vi "ButtonAutoRampStack.vi"(11 "Buttons":bool[](array[boolean])) -> ()   [LabVIEW 2014]
uses:
  LowerLiftAndOpenArms.ctl
  AutomationGlobals.vi
  ToteCount.vi
  Gantry/GantryGlobals.vi
panel:
  in  "Buttons 4":bool[](array[boolean])
  in  "Buttons 3":bool[](array[boolean])
  in  "Buttons 2":bool[](array[boolean])
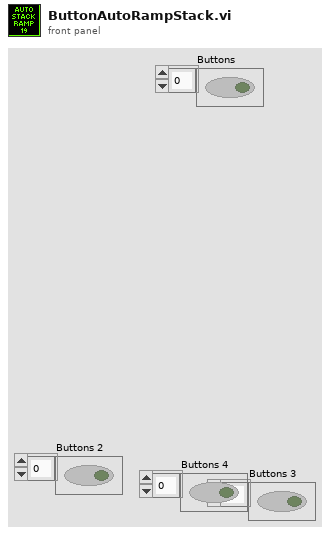
[diagram p1: front panel]
types:
  T1 = typedef "LowerLiftAndOpenArms.ctl" = enum16{"WaitingForInput", "LowerLift", "OpenArms", "LowerLiftMore", "CloseArms", "RaiseLift", "StopArms"}
  T2 = typedef "WPI_SwitchDevRef.ctl" = cluster{"DevStatus":errorcluster, "DIO Channel":T3, "Controller":T4, "CntIndex":T5, "Normally Closed":bool}
  T3 = typedef "FPGA_DIOChannel.ctl" = enum8{"DIO 0", "DIO 1", "DIO 2", "DIO 3", "DIO 4", "DIO 5", "DIO 6", "DIO 7", "DIO 8", "DIO 9", "DIO MXP 0", "DIO MXP 1", "DIO MXP 2", "DIO MXP 3", "DIO MXP 4", "DIO MXP 5", "DIO MXP 6", "DIO MXP 7", "DIO MXP 8", "DIO MXP 9", "DIO MXP 10", "DIO MXP 11", "DIO MXP 12", "DIO MXP 13", "DIO MXP 14", "DIO MXP 15", "Invalid"}
  T4 = typedef "FPGA_TypedefDigitalModule.ctl" = enum16{"Controller 1"}
  T5 = typedef "FPGA_CounterCtrSystemIndex.ctl" = enum8{"Ctr 0", "Ctr 1", "Ctr 2", "Ctr 3", "Ctr 4", "Ctr 5", "Ctr 6", "Ctr 7", "Invalid"}
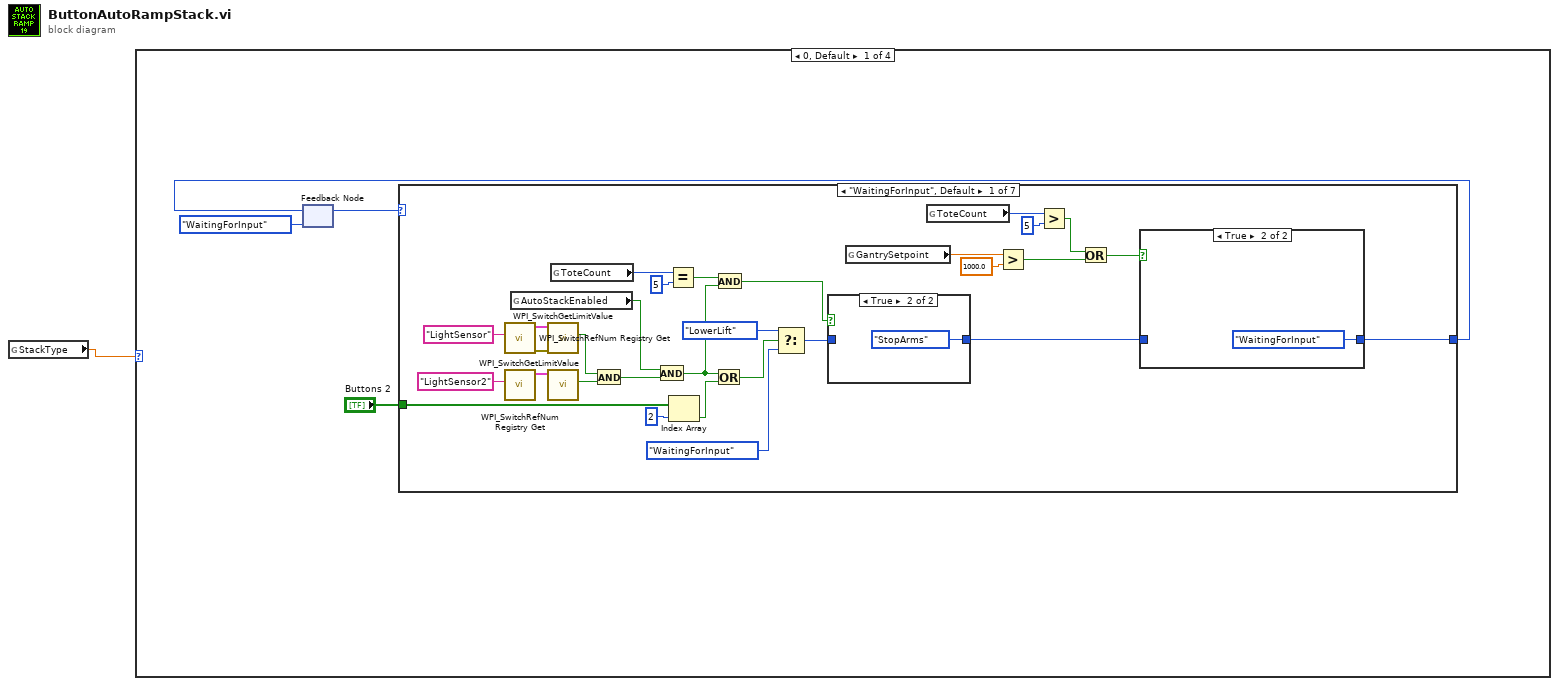
[diagram p0: block diagram]
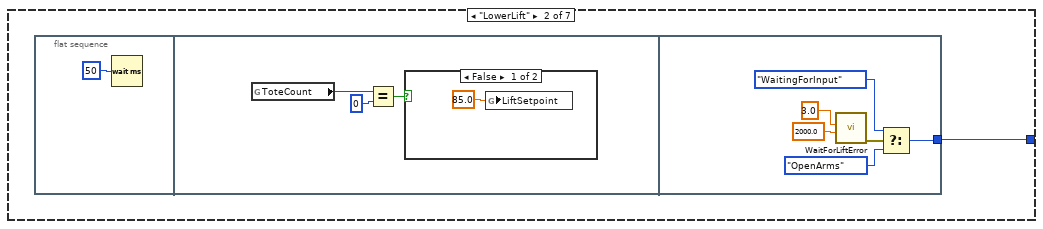
[diagram p4: hidden frame]
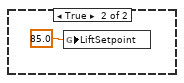
[diagram p5: hidden frame]
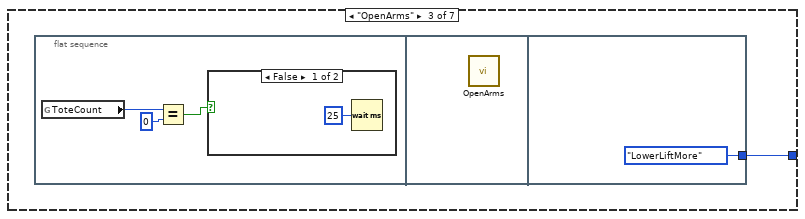
[diagram p6: hidden frame]
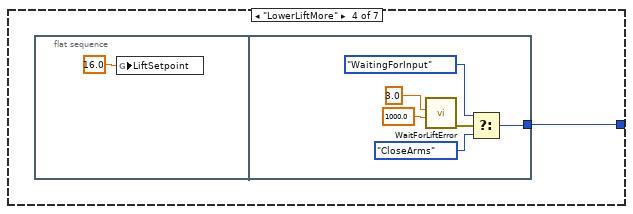
[diagram p8: hidden frame]
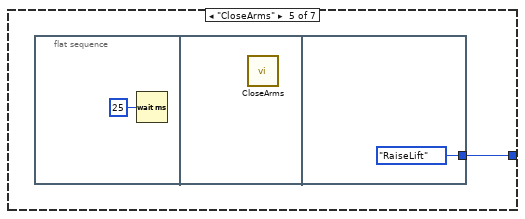
[diagram p9: hidden frame]
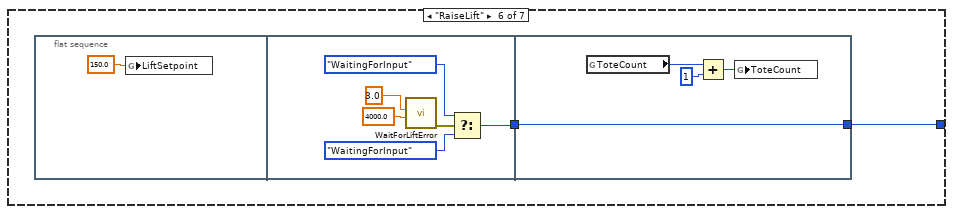
[diagram p10: hidden frame]
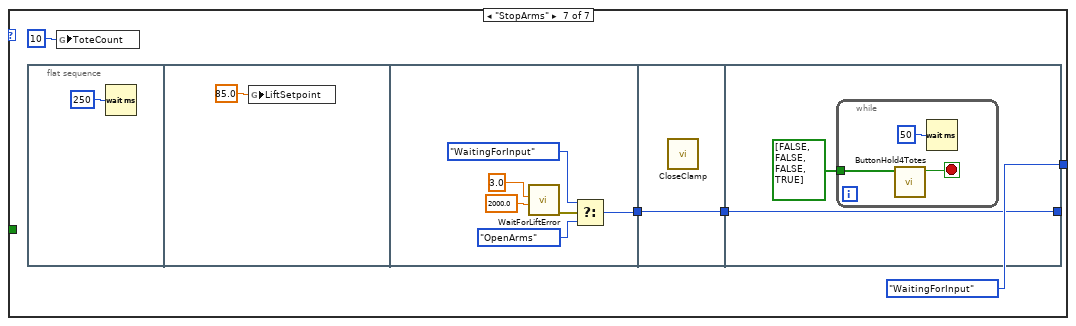
[diagram p11: hidden frame]
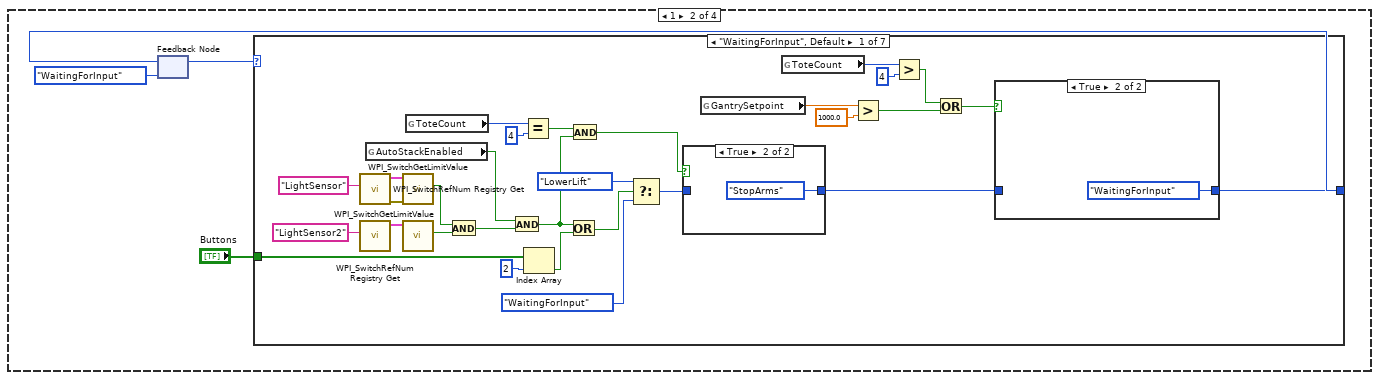
[diagram p12: hidden frame]
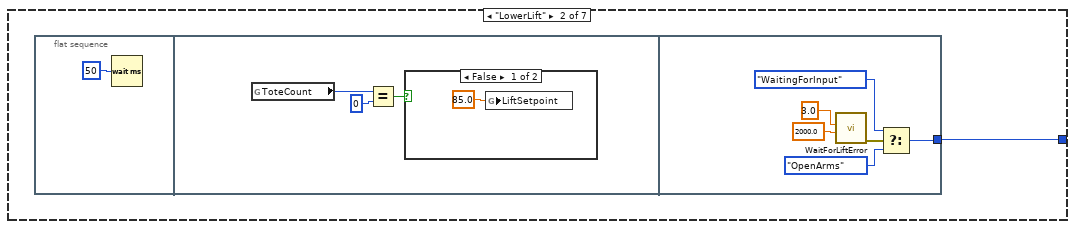
[diagram p15: hidden frame]
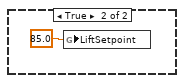
[diagram p16: hidden frame]
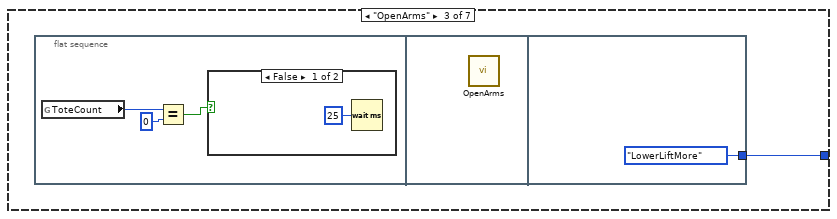
[diagram p17: hidden frame]
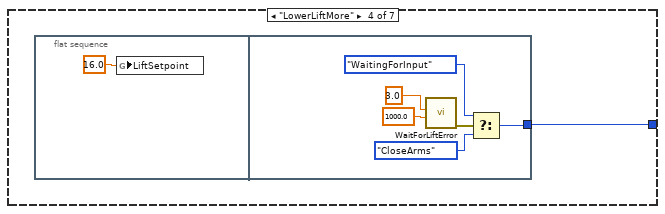
[diagram p19: hidden frame]
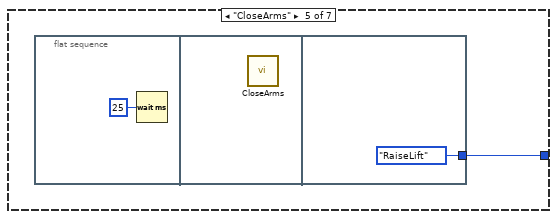
[diagram p20: hidden frame]
diagram:
  n1 = global read "AutomationGlobals.vi" "StackType"() -> (w1:dbl)
  n2 = case shown="0, Default" w1 {
    frame 0, Default {
      n3 = feedback #1(LowerLiftAndOpenArms."WaitingForInput" ("LowerAndOpen")) -> (w2:T1)
      n4 = case shown="\"WaitingForInput\", Default" w2 {
        tunnel: [w20 w40 w53 w59 w67 w71 LowerLiftAndOpenArms."WaitingForInput" ("LowerAndOpen")] -> w5
        tunnel: "Buttons 2" -> [w34 _ _ _ _ _ _]
        frame "WaitingForInput", Default {
          n5 = call <vilib>:"WPI_SwitchRefNum Registry Get.vi"("refnum name"="LightSensor") -> ("error out"=w31:errorcluster, "SwitchDevRef"=w32:T2)  [unwired: 9 in]
          n6 = call <vilib>:"WPI_SwitchRefNum Registry Get.vi"("refnum name"="LightSensor2") -> ("SwitchDevRef"=w9:T2)  [unwired: 9 in, 1 out]
          n7 = global read "AutomationGlobals.vi" "AutoStackEnabled"() -> (w13:bool)
          n8 = call <vilib>:"WPI_SwitchGetLimitValue.vi"("error in (no error)"=w31, "SwitchDevRef"=w32) -> ("Switch Pressed"=w7:bool)  [unwired: 7 in, 2 out]
          n9 = call <vilib>:"WPI_SwitchGetLimitValue.vi"("SwitchDevRef"=w9) -> ("Switch Pressed"=w8:bool)  [unwired: 8 in, 2 out]
          n10 = global read "ToteCount.vi" "ToteCount"() -> (w26:i32)
          n11 = And(x=w7, y=w8) -> (x .and. y?=w6:bool)
          n12 = And(x=w13, y=w6) -> (x .and. y?=w12:bool)
          n13 = Equal?(x=w26, y=5) -> (x = y?=w19:bool)
          n14 = Index Array(array=w34, index=2) -> (element=w28:bool)
          n15 = Or(x=w12, y=w28) -> (x .or. y?=w27:bool)
          n16 = And(x=w19, y=w12) -> (x .and. y?=w15:bool)
          n17 = Select(t=LowerLiftAndOpenArms."LowerLift" ("LowerAndOpen"), s=w27, f=LowerLiftAndOpenArms."WaitingForInput" ("LowerAndOpen")) -> (s? t:f=w24:T1)
          n18 = case shown="True" w15 {
            tunnel: w24 -> [w38 _]
            tunnel: [w38 LowerLiftAndOpenArms."StopArms" ("LowerAndOpen")] -> w21
            frame False {
            }
            frame True {
            }
          }
          n19 = global read "GantryGlobals.vi" "GantrySetpoint"() -> (w17:dbl)
          n20 = global read "ToteCount.vi" "ToteCount"() -> (w23:i32)
          n21 = Greater?(x=w17, y=1000.0) -> (0:w14:bool)
          n22 = Greater?(x=w23, y=5) -> (0:w16:bool)
          n23 = Or(x=w16, y=w14) -> (x .or. y?=w11:bool)
          n24 = case shown="True" w11 {
            tunnel: w21 -> [w36 _]
            tunnel: [w36 LowerLiftAndOpenArms."WaitingForInput" ("LowerAndOpen")] -> w20
            frame False {
            }
            frame True {
            }
          }
        }
        frame "LowerLift" {
          n25 = flat-sequence {
            tunnel: [w47] -> w40
            frame #0 {
              n26 = Wait (ms)(milliseconds to wait=u32 50) -> ()  [unwired: 1 out]
            }
            frame #1 {
              n27 = global read "ToteCount.vi" "ToteCount"() -> (w44:i32)
              n28 = Equal?(x=w44, y=0) -> (x = y?=w42:bool)
              n29 = case shown="False" w42 {
                frame False {
                  n30 = global write "GantryGlobals.vi" "LiftSetpoint"(85.0 ("LiftSetpoint")) -> ()
                }
                frame True {
                  n31 = global write "GantryGlobals.vi" "LiftSetpoint"(85.0 ("LiftSetpoint")) -> ()
                }
              }
            }
            frame #2 {
              n32 = call "WaitForLiftError.vi"("Timeout (ms)"=2000.0, "AllowedError"=3.0) -> ("error out"=w50:errorcluster)  [unwired: 9 in]
              n33 = Select(t=LowerLiftAndOpenArms."WaitingForInput" ("LowerAndOpen"), s=w50, f=LowerLiftAndOpenArms."OpenArms" ("LowerAndOpen")) -> (s? t:f=w47:T1)
            }
          }
        }
        frame "OpenArms" {
          n34 = flat-sequence {
            tunnel: [LowerLiftAndOpenArms."LowerLiftMore" ("LowerAndOpen")] -> w53
            frame #0 {
              n35 = global read "ToteCount.vi" "ToteCount"() -> (w56:i32)
              n36 = Equal?(x=w56, y=0) -> (x = y?=w54:bool)
              n37 = case shown="False" w54 {
                frame False {
                  n38 = Wait (ms)(milliseconds to wait=u32 25) -> ()  [unwired: 1 out]
                }
                frame True {
                }
              }
            }
            frame #1 {
              n39 = call "OpenArms.vi"() -> ()  [unwired: 12 in]
            }
            frame #2 {
            }
          }
        }
        frame "LowerLiftMore" {
          n40 = flat-sequence {
            tunnel: [w61] -> w59
            frame #0 {
              n41 = global write "GantryGlobals.vi" "LiftSetpoint"(16.0 ("LiftSetpoint")) -> ()
            }
            frame #1 {
              n42 = call "WaitForLiftError.vi"("Timeout (ms)"=1000.0, "AllowedError"=3.0) -> ("error out"=w64:errorcluster)  [unwired: 9 in]
              n43 = Select(t=LowerLiftAndOpenArms."WaitingForInput" ("LowerAndOpen"), s=w64, f=LowerLiftAndOpenArms."CloseArms" ("LowerAndOpen")) -> (s? t:f=w61:T1)
            }
          }
        }
        frame "CloseArms" {
          n44 = flat-sequence {
            tunnel: [LowerLiftAndOpenArms."RaiseLift" ("LowerAndOpen")] -> w67
            frame #0 {
              n45 = Wait (ms)(milliseconds to wait=u32 25) -> ()  [unwired: 1 out]
            }
            frame #1 {
              n46 = call "CloseArms.vi"() -> ()  [unwired: 12 in]
            }
            frame #2 {
            }
          }
        }
        frame "RaiseLift" {
          n47 = flat-sequence {
            tunnel: [w73] -> w70
            tunnel: [w82] -> w71
            tunnel: w70 -> [w82]
            frame #0 {
              n48 = global write "GantryGlobals.vi" "LiftSetpoint"(150.0 ("LiftSetpoint")) -> ()
            }
            frame #1 {
              n49 = call "WaitForLiftError.vi"("Timeout (ms)"=4000.0, "AllowedError"=3.0) -> ("error out"=w76:errorcluster)  [unwired: 9 in]
              n50 = Select(t=LowerLiftAndOpenArms."WaitingForInput" ("LowerAndOpen"), s=w76, f=LowerLiftAndOpenArms."WaitingForInput" ("LowerAndOpen")) -> (s? t:f=w73:T1)
            }
            frame #2 {
              n51 = global read "ToteCount.vi" "ToteCount"() -> (w81:i32)
              n52 = Add(x=w81, y=1) -> (x+y=w79:i32)
              n53 = global write "ToteCount.vi" "ToteCount"(w79) -> ()
            }
          }
        }
        frame "StopArms" {
          n54 = flat-sequence {
            tunnel: [w89] -> w84
            tunnel: w84 -> [w95]
            tunnel: [w95] -> w83
            tunnel: [w97] -> _
            tunnel: w83 -> [w97]
            frame #0 {
              n55 = Wait (ms)(milliseconds to wait=u32 250) -> ()  [unwired: 1 out]
            }
            frame #1 {
              n56 = global write "GantryGlobals.vi" "LiftSetpoint"(85.0 ("LiftSetpoint")) -> ()
            }
            frame #2 {
              n57 = call "WaitForLiftError.vi"("Timeout (ms)"=2000.0, "AllowedError"=3.0) -> ("error out"=w92:errorcluster)  [unwired: 9 in]
              n58 = Select(t=LowerLiftAndOpenArms."WaitingForInput" ("LowerAndOpen"), s=w92, f=LowerLiftAndOpenArms."OpenArms" ("LowerAndOpen")) -> (s? t:f=w89:T1)
            }
            frame #3 {
              n59 = call "CloseClamp.vi"() -> ()  [unwired: 12 in]
            }
            frame #4 {
              n60 = while {
                tunnel: bool[] [FALSE, FALSE, FALSE, TRUE] ("Buttons") -> [w100]
                stop <- w99 stop-if-true
                n61 = call "ButtonHold4Totes.vi"("Buttons"=w100) -> ("Boolean"=w99:bool)  [unwired: 10 in]
                n62 = Wait (ms)(milliseconds to wait=u32 50) -> ()  [unwired: 1 out]
              }
            }
          }
          n63 = global write "ToteCount.vi" "ToteCount"(10 ("ToteCount")) -> ()
        }
      }
      n64 = feedback-in #1(w5) -> ()
    }
    frame 1 {
      n65 = feedback #2(LowerLiftAndOpenArms."WaitingForInput" ("LowerAndOpen")) -> (w101:T1)
      n66 = case shown="\"WaitingForInput\", Default" w101 {
        tunnel: [w119 w139 w152 w158 w166 w170 LowerLiftAndOpenArms."WaitingForInput" ("LowerAndOpen")] -> w104
        tunnel: "Buttons" -> [w133 _ _ _ _ _ _]
        frame "WaitingForInput", Default {
          n67 = call <vilib>:"WPI_SwitchRefNum Registry Get.vi"("refnum name"="LightSensor") -> ("error out"=w130:errorcluster, "SwitchDevRef"=w131:T2)  [unwired: 9 in]
          n68 = call <vilib>:"WPI_SwitchRefNum Registry Get.vi"("refnum name"="LightSensor2") -> ("SwitchDevRef"=w108:T2)  [unwired: 9 in, 1 out]
          n69 = global read "AutomationGlobals.vi" "AutoStackEnabled"() -> (w112:bool)
          n70 = call <vilib>:"WPI_SwitchGetLimitValue.vi"("error in (no error)"=w130, "SwitchDevRef"=w131) -> ("Switch Pressed"=w106:bool)  [unwired: 7 in, 2 out]
          n71 = call <vilib>:"WPI_SwitchGetLimitValue.vi"("SwitchDevRef"=w108) -> ("Switch Pressed"=w107:bool)  [unwired: 8 in, 2 out]
          n72 = global read "ToteCount.vi" "ToteCount"() -> (w125:i32)
          n73 = And(x=w106, y=w107) -> (x .and. y?=w105:bool)
          n74 = And(x=w112, y=w105) -> (x .and. y?=w111:bool)
          n75 = Equal?(x=w125, y=4) -> (x = y?=w118:bool)
          n76 = Index Array(array=w133, index=2) -> (element=w127:bool)
          n77 = Or(x=w111, y=w127) -> (x .or. y?=w126:bool)
          n78 = And(x=w118, y=w111) -> (x .and. y?=w114:bool)
          n79 = Select(t=LowerLiftAndOpenArms."LowerLift" ("LowerAndOpen"), s=w126, f=LowerLiftAndOpenArms."WaitingForInput" ("LowerAndOpen")) -> (s? t:f=w123:T1)
          n80 = case shown="True" w114 {
            tunnel: w123 -> [w137 _]
            tunnel: [w137 LowerLiftAndOpenArms."StopArms" ("LowerAndOpen")] -> w120
            frame False {
            }
            frame True {
            }
          }
          n81 = global read "GantryGlobals.vi" "GantrySetpoint"() -> (w116:dbl)
          n82 = global read "ToteCount.vi" "ToteCount"() -> (w122:i32)
          n83 = Greater?(x=w116, y=1000.0) -> (0:w113:bool)
          n84 = Greater?(x=w122, y=4) -> (0:w115:bool)
          n85 = Or(x=w115, y=w113) -> (x .or. y?=w110:bool)
          n86 = case shown="True" w110 {
            tunnel: w120 -> [w135 _]
            tunnel: [w135 LowerLiftAndOpenArms."WaitingForInput" ("LowerAndOpen")] -> w119
            frame False {
            }
            frame True {
            }
          }
        }
        frame "LowerLift" {
          n87 = flat-sequence {
            tunnel: [w146] -> w139
            frame #0 {
              n88 = Wait (ms)(milliseconds to wait=u32 50) -> ()  [unwired: 1 out]
            }
            frame #1 {
              n89 = global read "ToteCount.vi" "ToteCount"() -> (w143:i32)
              n90 = Equal?(x=w143, y=0) -> (x = y?=w141:bool)
              n91 = case shown="False" w141 {
                frame False {
                  n92 = global write "GantryGlobals.vi" "LiftSetpoint"(85.0 ("LiftSetpoint")) -> ()
                }
                frame True {
                  n93 = global write "GantryGlobals.vi" "LiftSetpoint"(85.0 ("LiftSetpoint")) -> ()
                }
              }
            }
            frame #2 {
              n94 = call "WaitForLiftError.vi"("Timeout (ms)"=2000.0, "AllowedError"=3.0) -> ("error out"=w149:errorcluster)  [unwired: 9 in]
              n95 = Select(t=LowerLiftAndOpenArms."WaitingForInput" ("LowerAndOpen"), s=w149, f=LowerLiftAndOpenArms."OpenArms" ("LowerAndOpen")) -> (s? t:f=w146:T1)
            }
          }
        }
        frame "OpenArms" {
          n96 = flat-sequence {
            tunnel: [LowerLiftAndOpenArms."LowerLiftMore" ("LowerAndOpen")] -> w152
            frame #0 {
              n97 = global read "ToteCount.vi" "ToteCount"() -> (w155:i32)
              n98 = Equal?(x=w155, y=0) -> (x = y?=w153:bool)
              n99 = case shown="False" w153 {
                frame False {
                  n100 = Wait (ms)(milliseconds to wait=u32 25) -> ()  [unwired: 1 out]
                }
                frame True {
                }
              }
            }
            frame #1 {
              n101 = call "OpenArms.vi"() -> ()  [unwired: 12 in]
            }
            frame #2 {
            }
          }
        }
        frame "LowerLiftMore" {
          n102 = flat-sequence {
            tunnel: [w160] -> w158
            frame #0 {
              n103 = global write "GantryGlobals.vi" "LiftSetpoint"(16.0 ("LiftSetpoint")) -> ()
            }
            frame #1 {
              n104 = call "WaitForLiftError.vi"("Timeout (ms)"=1000.0, "AllowedError"=3.0) -> ("error out"=w163:errorcluster)  [unwired: 9 in]
              n105 = Select(t=LowerLiftAndOpenArms."WaitingForInput" ("LowerAndOpen"), s=w163, f=LowerLiftAndOpenArms."CloseArms" ("LowerAndOpen")) -> (s? t:f=w160:T1)
            }
          }
        }
        frame "CloseArms" {
          n106 = flat-sequence {
            tunnel: [LowerLiftAndOpenArms."RaiseLift" ("LowerAndOpen")] -> w166
            frame #0 {
              n107 = Wait (ms)(milliseconds to wait=u32 25) -> ()  [unwired: 1 out]
            }
            frame #1 {
              n108 = call "CloseArms.vi"() -> ()  [unwired: 12 in]
            }
            frame #2 {
            }
          }
        }
        frame "RaiseLift" {
          n109 = flat-sequence {
            tunnel: [w172] -> w169
            tunnel: [w181] -> w170
            tunnel: w169 -> [w181]
            frame #0 {
              n110 = global write "GantryGlobals.vi" "LiftSetpoint"(150.0 ("LiftSetpoint")) -> ()
            }
            frame #1 {
              n111 = call "WaitForLiftError.vi"("Timeout (ms)"=4000.0, "AllowedError"=3.0) -> ("error out"=w175:errorcluster)  [unwired: 9 in]
              n112 = Select(t=LowerLiftAndOpenArms."WaitingForInput" ("LowerAndOpen"), s=w175, f=LowerLiftAndOpenArms."WaitingForInput" ("LowerAndOpen")) -> (s? t:f=w172:T1)
            }
            frame #2 {
              n113 = global read "ToteCount.vi" "ToteCount"() -> (w180:i32)
              n114 = Add(x=w180, y=1) -> (x+y=w178:i32)
              n115 = global write "ToteCount.vi" "ToteCount"(w178) -> ()
            }
          }
        }
        frame "StopArms" {
          n116 = global write "ToteCount.vi" "ToteCount"(10 ("ToteCount")) -> ()
          n117 = flat-sequence {
            tunnel: [w188] -> w183
            tunnel: w183 -> [w194]
            tunnel: [w194] -> w182
            tunnel: [w196] -> _
            tunnel: w182 -> [w196]
            frame #0 {
              n118 = Wait (ms)(milliseconds to wait=u32 250) -> ()  [unwired: 1 out]
            }
            frame #1 {
              n119 = global write "GantryGlobals.vi" "LiftSetpoint"(85.0 ("LiftSetpoint")) -> ()
            }
            frame #2 {
              n120 = call "WaitForLiftError.vi"("Timeout (ms)"=2000.0, "AllowedError"=3.0) -> ("error out"=w191:errorcluster)  [unwired: 9 in]
              n121 = Select(t=LowerLiftAndOpenArms."WaitingForInput" ("LowerAndOpen"), s=w191, f=LowerLiftAndOpenArms."OpenArms" ("LowerAndOpen")) -> (s? t:f=w188:T1)
            }
            frame #3 {
              n122 = call "CloseClamp.vi"() -> ()  [unwired: 12 in]
            }
            frame #4 {
              n123 = while {
                tunnel: bool[] [FALSE, FALSE, FALSE, TRUE] ("Buttons") -> [w198]
                stop <- w197 stop-if-true
                n124 = call "ButtonHold4Totes.vi"("Buttons"=w198) -> ("Boolean"=w197:bool)  [unwired: 10 in]
                n125 = Wait (ms)(milliseconds to wait=u32 50) -> ()  [unwired: 1 out]
              }
            }
          }
        }
      }
      n126 = feedback-in #2(w104) -> ()
    }
    frame 2 {
      n127 = feedback #3(LowerLiftAndOpenArms."WaitingForInput" ("LowerAndOpen")) -> (w200:T1)
      n128 = case shown="\"WaitingForInput\", Default" w200 {
        tunnel: [w221 w236 w245 w251 w259 w263 LowerLiftAndOpenArms."WaitingForInput" ("LowerAndOpen")] -> w203
        tunnel: "Buttons 3" -> [w230 _ _ _ _ _ _]
        frame "WaitingForInput", Default {
          n129 = call <vilib>:"WPI_SwitchRefNum Registry Get.vi"("refnum name"="LightSensor") -> ("error out"=w227:errorcluster, "SwitchDevRef"=w228:T2)  [unwired: 9 in]
          n130 = call <vilib>:"WPI_SwitchRefNum Registry Get.vi"("refnum name"="LightSensor2") -> ("SwitchDevRef"=w211:T2)  [unwired: 9 in, 1 out]
          n131 = global read "AutomationGlobals.vi" "AutoStackEnabled"() -> (w214:bool)
          n132 = call <vilib>:"WPI_SwitchGetLimitValue.vi"("error in (no error)"=w227, "SwitchDevRef"=w228) -> ("Switch Pressed"=w209:bool)  [unwired: 7 in, 2 out]
          n133 = call <vilib>:"WPI_SwitchGetLimitValue.vi"("SwitchDevRef"=w211) -> ("Switch Pressed"=w210:bool)  [unwired: 8 in, 2 out]
          n134 = global read "ToteCount.vi" "ToteCount"() -> (w226:i32)
          n135 = And(x=w209, y=w210) -> (x .and. y?=w208:bool)
          n136 = And(x=w214, y=w208) -> ()  [unwired: 1 out]
          n137 = Equal?(x=w226, y=3) -> (x = y?=w220:bool)
          n138 = Index Array(array=w230, index=2) -> (element=w204:bool)
          n139 = And(x=w220, y=w204) -> (x .and. y?=w216:bool)
          n140 = Select(t=LowerLiftAndOpenArms."LowerLift" ("LowerAndOpen"), s=w204, f=LowerLiftAndOpenArms."WaitingForInput" ("LowerAndOpen")) -> (s? t:f=w205:T1)
          n141 = case shown="False" w216 {
            tunnel: [w234 LowerLiftAndOpenArms."StopArms" ("LowerAndOpen")] -> w222
            tunnel: w205 -> [w234 _]
            frame False {
            }
            frame True {
            }
          }
          n142 = global read "GantryGlobals.vi" "GantrySetpoint"() -> (w218:dbl)
          n143 = global read "ToteCount.vi" "ToteCount"() -> (w224:i32)
          n144 = Greater?(x=w218, y=1000.0) -> (0:w215:bool)
          n145 = Greater?(x=w224, y=3) -> (0:w217:bool)
          n146 = Or(x=w217, y=w215) -> (x .or. y?=w213:bool)
          n147 = case shown="False" w213 {
            tunnel: w222 -> [w232 _]
            tunnel: [w232 LowerLiftAndOpenArms."WaitingForInput" ("LowerAndOpen")] -> w221
            frame False {
            }
            frame True {
            }
          }
        }
        frame "LowerLift" {
          n148 = flat-sequence {
            tunnel: [w239] -> w236
            frame #0 {
              n149 = Wait (ms)(milliseconds to wait=u32 50) -> ()  [unwired: 1 out]
            }
            frame #1 {
              n150 = global write "GantryGlobals.vi" "LiftSetpoint"(135.0 ("LiftSetpoint")) -> ()
            }
            frame #2 {
              n151 = call "WaitForLiftError.vi"("Timeout (ms)"=2000.0, "AllowedError"=3.0) -> ("error out"=w242:errorcluster)  [unwired: 9 in]
              n152 = Select(t=LowerLiftAndOpenArms."WaitingForInput" ("LowerAndOpen"), s=w242, f=LowerLiftAndOpenArms."OpenArms" ("LowerAndOpen")) -> (s? t:f=w239:T1)
            }
          }
        }
        frame "OpenArms" {
          n153 = flat-sequence {
            tunnel: [LowerLiftAndOpenArms."LowerLiftMore" ("LowerAndOpen")] -> w245
            frame #0 {
              n154 = global read "ToteCount.vi" "ToteCount"() -> (w248:i32)
              n155 = Equal?(x=w248, y=0) -> (x = y?=w246:bool)
              n156 = case shown="False" w246 {
                frame False {
                  n157 = Wait (ms)(milliseconds to wait=u32 25) -> ()  [unwired: 1 out]
                }
                frame True {
                }
              }
            }
            frame #1 {
              n158 = call "OpenArms.vi"() -> ()  [unwired: 12 in]
            }
            frame #2 {
            }
          }
        }
        frame "LowerLiftMore" {
          n159 = flat-sequence {
            tunnel: [w253] -> w251
            frame #0 {
              n160 = global write "GantryGlobals.vi" "LiftSetpoint"(85.0 ("LiftSetpoint")) -> ()
            }
            frame #1 {
              n161 = call "WaitForLiftError.vi"("Timeout (ms)"=1000.0, "AllowedError"=3.0) -> ("error out"=w256:errorcluster)  [unwired: 9 in]
              n162 = Select(t=LowerLiftAndOpenArms."WaitingForInput" ("LowerAndOpen"), s=w256, f=LowerLiftAndOpenArms."CloseArms" ("LowerAndOpen")) -> (s? t:f=w253:T1)
            }
          }
        }
        frame "CloseArms" {
          n163 = flat-sequence {
            tunnel: [LowerLiftAndOpenArms."RaiseLift" ("LowerAndOpen")] -> w259
            frame #0 {
              n164 = Wait (ms)(milliseconds to wait=u32 25) -> ()  [unwired: 1 out]
            }
            frame #1 {
              n165 = call "CloseArms.vi"() -> ()  [unwired: 12 in]
            }
            frame #2 {
            }
          }
        }
        frame "RaiseLift" {
          n166 = flat-sequence {
            tunnel: [w265] -> w262
            tunnel: [w274] -> w263
            tunnel: w262 -> [w274]
            frame #0 {
              n167 = global write "GantryGlobals.vi" "LiftSetpoint"(200.0 ("LiftSetpoint")) -> ()
            }
            frame #1 {
              n168 = call "WaitForLiftError.vi"("Timeout (ms)"=4000.0, "AllowedError"=3.0) -> ("error out"=w268:errorcluster)  [unwired: 9 in]
              n169 = Select(t=LowerLiftAndOpenArms."WaitingForInput" ("LowerAndOpen"), s=w268, f=LowerLiftAndOpenArms."WaitingForInput" ("LowerAndOpen")) -> (s? t:f=w265:T1)
            }
            frame #2 {
              n170 = global read "ToteCount.vi" "ToteCount"() -> (w273:i32)
              n171 = Add(x=w273, y=1) -> (x+y=w271:i32)
              n172 = global write "ToteCount.vi" "ToteCount"(w271) -> ()
            }
          }
        }
        frame "StopArms" {
          n173 = global write "ToteCount.vi" "ToteCount"(10 ("ToteCount")) -> ()
          n174 = flat-sequence {
            tunnel: [w281] -> w276
            tunnel: w276 -> [w287]
            tunnel: [w287] -> w275
            tunnel: [w289] -> _
            tunnel: w275 -> [w289]
            frame #0 {
              n175 = Wait (ms)(milliseconds to wait=u32 250) -> ()  [unwired: 1 out]
            }
            frame #1 {
              n176 = global write "GantryGlobals.vi" "LiftSetpoint"(85.0 ("LiftSetpoint")) -> ()
            }
            frame #2 {
              n177 = call "WaitForLiftError.vi"("Timeout (ms)"=2000.0, "AllowedError"=3.0) -> ("error out"=w284:errorcluster)  [unwired: 9 in]
              n178 = Select(t=LowerLiftAndOpenArms."WaitingForInput" ("LowerAndOpen"), s=w284, f=LowerLiftAndOpenArms."OpenArms" ("LowerAndOpen")) -> (s? t:f=w281:T1)
            }
            frame #3 {
              n179 = call "CloseClamp.vi"() -> ()  [unwired: 12 in]
            }
            frame #4 {
              n180 = while {
                tunnel: bool[] [FALSE, FALSE, FALSE, TRUE] ("Buttons") -> [w290]
                stop <- w291 stop-if-true
                n181 = call "ButtonHold4Totes.vi"("Buttons"=w290) -> ("Boolean"=w291:bool)  [unwired: 10 in]
                n182 = Wait (ms)(milliseconds to wait=u32 50) -> ()  [unwired: 1 out]
              }
            }
          }
        }
      }
      n183 = feedback-in #3(w203) -> ()
    }
    frame 3 {
      n184 = feedback #4(LowerLiftAndOpenArms."WaitingForInput" ("LowerAndOpen")) -> (w293:T1)
      n185 = case shown="\"WaitingForInput\", Default" w293 {
        tunnel: [w314 w329 w342 w348 w356 w360 LowerLiftAndOpenArms."WaitingForInput" ("LowerAndOpen")] -> w296
        tunnel: "Buttons 4" -> [w323 _ _ _ _ _ _]
        frame "WaitingForInput", Default {
          n186 = call <vilib>:"WPI_SwitchRefNum Registry Get.vi"("refnum name"="LightSensor") -> ("error out"=w320:errorcluster, "SwitchDevRef"=w321:T2)  [unwired: 9 in]
          n187 = call <vilib>:"WPI_SwitchRefNum Registry Get.vi"("refnum name"="LightSensor2") -> ("SwitchDevRef"=w304:T2)  [unwired: 9 in, 1 out]
          n188 = global read "AutomationGlobals.vi" "AutoStackEnabled"() -> (w307:bool)
          n189 = call <vilib>:"WPI_SwitchGetLimitValue.vi"("error in (no error)"=w320, "SwitchDevRef"=w321) -> ("Switch Pressed"=w302:bool)  [unwired: 7 in, 2 out]
          n190 = call <vilib>:"WPI_SwitchGetLimitValue.vi"("SwitchDevRef"=w304) -> ("Switch Pressed"=w303:bool)  [unwired: 8 in, 2 out]
          n191 = global read "ToteCount.vi" "ToteCount"() -> (w319:i32)
          n192 = And(x=w302, y=w303) -> (x .and. y?=w301:bool)
          n193 = And(x=w307, y=w301) -> ()  [unwired: 1 out]
          n194 = Equal?(x=w319, y=4) -> (x = y?=w313:bool)
          n195 = Index Array(array=w323, index=2) -> (element=w297:bool)
          n196 = And(x=w313, y=w297) -> (x .and. y?=w309:bool)
          n197 = Select(t=LowerLiftAndOpenArms."LowerLift" ("LowerAndOpen"), s=w297, f=LowerLiftAndOpenArms."WaitingForInput" ("LowerAndOpen")) -> (s? t:f=w298:T1)
          n198 = case shown="True" w309 {
            tunnel: [w327 LowerLiftAndOpenArms."StopArms" ("LowerAndOpen")] -> w315
            tunnel: w298 -> [w327 _]
            frame False {
            }
            frame True {
            }
          }
          n199 = global read "GantryGlobals.vi" "GantrySetpoint"() -> (w311:dbl)
          n200 = global read "ToteCount.vi" "ToteCount"() -> (w317:i32)
          n201 = Greater?(x=w311, y=1000.0) -> (0:w308:bool)
          n202 = Greater?(x=w317, y=4) -> (0:w310:bool)
          n203 = Or(x=w310, y=w308) -> (x .or. y?=w306:bool)
          n204 = case shown="True" w306 {
            tunnel: w315 -> [w325 _]
            tunnel: [w325 LowerLiftAndOpenArms."WaitingForInput" ("LowerAndOpen")] -> w314
            frame False {
            }
            frame True {
            }
          }
        }
        frame "LowerLift" {
          n205 = flat-sequence {
            tunnel: [w336] -> w329
            frame #0 {
              n206 = Wait (ms)(milliseconds to wait=u32 50) -> ()  [unwired: 1 out]
            }
            frame #1 {
              n207 = global read "ToteCount.vi" "ToteCount"() -> (w333:i32)
              n208 = Equal?(x=w333, y=0) -> (x = y?=w331:bool)
              n209 = case shown="False" w331 {
                frame False {
                  n210 = global write "GantryGlobals.vi" "LiftSetpoint"(135.0 ("LiftSetpoint")) -> ()
                }
                frame True {
                  n211 = global write "GantryGlobals.vi" "LiftSetpoint"(85.0 ("LiftSetpoint")) -> ()
                }
              }
            }
            frame #2 {
              n212 = call "WaitForLiftError.vi"("Timeout (ms)"=2000.0, "AllowedError"=3.0) -> ("error out"=w339:errorcluster)  [unwired: 9 in]
              n213 = Select(t=LowerLiftAndOpenArms."WaitingForInput" ("LowerAndOpen"), s=w339, f=LowerLiftAndOpenArms."OpenArms" ("LowerAndOpen")) -> (s? t:f=w336:T1)
            }
          }
        }
        frame "OpenArms" {
          n214 = flat-sequence {
            tunnel: [LowerLiftAndOpenArms."LowerLiftMore" ("LowerAndOpen")] -> w342
            frame #0 {
              n215 = global read "ToteCount.vi" "ToteCount"() -> (w345:i32)
              n216 = Equal?(x=w345, y=0) -> (x = y?=w343:bool)
              n217 = case shown="False" w343 {
                frame False {
                  n218 = Wait (ms)(milliseconds to wait=u32 25) -> ()  [unwired: 1 out]
                }
                frame True {
                }
              }
            }
            frame #1 {
              n219 = call "OpenArms.vi"() -> ()  [unwired: 12 in]
            }
            frame #2 {
            }
          }
        }
        frame "LowerLiftMore" {
          n220 = flat-sequence {
            tunnel: [w350] -> w348
            frame #0 {
              n221 = global write "GantryGlobals.vi" "LiftSetpoint"(85.0 ("LiftSetpoint")) -> ()
            }
            frame #1 {
              n222 = call "WaitForLiftError.vi"("Timeout (ms)"=1000.0, "AllowedError"=3.0) -> ("error out"=w353:errorcluster)  [unwired: 9 in]
              n223 = Select(t=LowerLiftAndOpenArms."WaitingForInput" ("LowerAndOpen"), s=w353, f=LowerLiftAndOpenArms."CloseArms" ("LowerAndOpen")) -> (s? t:f=w350:T1)
            }
          }
        }
        frame "CloseArms" {
          n224 = flat-sequence {
            tunnel: [LowerLiftAndOpenArms."RaiseLift" ("LowerAndOpen")] -> w356
            frame #0 {
              n225 = Wait (ms)(milliseconds to wait=u32 25) -> ()  [unwired: 1 out]
            }
            frame #1 {
              n226 = call "CloseArms.vi"() -> ()  [unwired: 12 in]
            }
            frame #2 {
            }
          }
        }
        frame "RaiseLift" {
          n227 = flat-sequence {
            tunnel: [w362] -> w359
            tunnel: [w371] -> w360
            tunnel: w359 -> [w371]
            frame #0 {
              n228 = global write "GantryGlobals.vi" "LiftSetpoint"(200.0 ("LiftSetpoint")) -> ()
            }
            frame #1 {
              n229 = call "WaitForLiftError.vi"("Timeout (ms)"=4000.0, "AllowedError"=3.0) -> ("error out"=w365:errorcluster)  [unwired: 9 in]
              n230 = Select(t=LowerLiftAndOpenArms."WaitingForInput" ("LowerAndOpen"), s=w365, f=LowerLiftAndOpenArms."WaitingForInput" ("LowerAndOpen")) -> (s? t:f=w362:T1)
            }
            frame #2 {
              n231 = global read "ToteCount.vi" "ToteCount"() -> (w370:i32)
              n232 = Add(x=w370, y=1) -> (x+y=w368:i32)
              n233 = global write "ToteCount.vi" "ToteCount"(w368) -> ()
            }
          }
        }
        frame "StopArms" {
          n234 = flat-sequence {
            tunnel: [w378] -> w373
            tunnel: w373 -> [w384]
            tunnel: [w384] -> w372
            tunnel: [w386] -> _
            tunnel: w372 -> [w386]
            frame #0 {
              n235 = Wait (ms)(milliseconds to wait=u32 250) -> ()  [unwired: 1 out]
            }
            frame #1 {
              n236 = global write "GantryGlobals.vi" "LiftSetpoint"(85.0 ("LiftSetpoint")) -> ()
            }
            frame #2 {
              n237 = call "WaitForLiftError.vi"("Timeout (ms)"=2000.0, "AllowedError"=3.0) -> ("error out"=w381:errorcluster)  [unwired: 9 in]
              n238 = Select(t=LowerLiftAndOpenArms."WaitingForInput" ("LowerAndOpen"), s=w381, f=LowerLiftAndOpenArms."OpenArms" ("LowerAndOpen")) -> (s? t:f=w378:T1)
            }
            frame #3 {
              n239 = call "CloseClamp.vi"() -> ()  [unwired: 12 in]
            }
            frame #4 {
              n240 = while {
                tunnel: bool[] [FALSE, FALSE, FALSE] -> [w388]
                stop <- w387 stop-if-true
                n241 = call "ButtonHold4Totes.vi"("Buttons"=w388) -> ("Boolean"=w387:bool)  [unwired: 10 in]
                n242 = Wait (ms)(milliseconds to wait=u32 50) -> ()  [unwired: 1 out]
              }
            }
          }
          n243 = global write "ToteCount.vi" "ToteCount"(10 ("ToteCount")) -> ()
        }
      }
      n244 = feedback-in #4(w296) -> ()
    }
  }
